vi "PH_OceanOpticsSpectrometer.PC Set Integration Time.vi"(0 "VI in":refnum<vi>, 2 "Wanted Integration Time [ms]":u16, 5 "error in (no error)":errorcluster) -> (14 "VI out":refnum<vi>, 19 "error out":errorcluster)   [LabVIEW 2014, in "PH_OceanOpticsSpectrometer.lvlib"]
doc: "This VI sets the integration time."
uses:
  PH_OceanOpticsSpectrometer.lvlib
  CS_Core/BaseProcess/BaseProcess.lvlib
  PH_Basics/PH_Common/PH_Common.lvlib
  instr.lib/OceanOpticsSpectrometer/Ocean Optics 2000 4000 - Driver np.lvlib
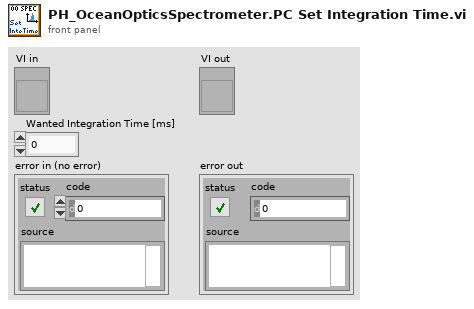
[diagram p1: front panel]
types:
  T1 = typedef "PH_OceanOpticsSpectrometer.lvlib/PH_OceanOpticsSpectrometer.i attribute.ctl" = cluster{"GUI Refs":cluster{"Delete":refnum<vi>, "Spectrum":refnum<vi>, "Display Width":refnum<vi>, "Display Center":refnum<vi>, "Save":refnum<vi>, "Integration time":refnum<vi>, "center wavelength":refnum<vi>, "width":refnum<vi>, "Wanted Trigger Mode":refnum<vi>, "Current Trigger Mode":refnum<vi>, "Trigger Info":refnum<vi>, "Model":refnum<vi>, "Driver":refnum<vi>, "Firmware":refnum<vi>}, "Display":cluster{"Width":dbl, "Center":dbl}, "VISA resource name":refnum<visa-resource-name>, "Integration time [ms]":cluster{"Current Value":u16, "Wanted Value":u16}, "Trigger":cluster{"Current value":T2, "Wanted value":T2}, "Default VISA Timeout":u32, "Last Data":cluster{"Wavelength Bins":dbl[], "Spectrum by Pixels":dbl[]}}
  T2 = typedef "PH_OceanOpticsSpectrometer.lvlib/PH_OceanOpticsSpectrometer.Trigger.ctl" = enum32{"External", "Normal"}
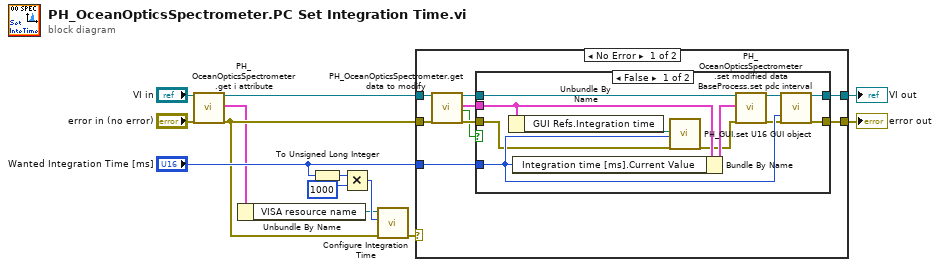
[diagram p0: block diagram]
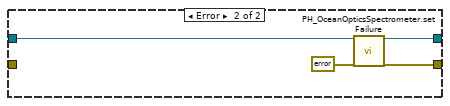
[diagram p3: hidden frame]
diagram:
  n1 = call "PH_OceanOpticsSpectrometer.get i attribute.vi"("i ref in"="VI in", "error in (no error)"="error in (no error)") -> ("i ref out"=w3:refnum<vi>, "i attribute"=w2:T1, "error out"=w5:errorcluster)  [unwired: 15 in]
  n2 = Unbundle By Name(w2) -> ("VISA resource name"=w1:refnum<visa-resource-name>)
  n3 = To Unsigned Long Integer(number="Wanted Integration Time [ms]") -> (unsigned 32bit integer=w13:u32)
  n4 = Multiply(x=w13, y=u32 1000 ("x")) -> (x*y=w9:u32)
  n5 = call "Configure Integration Time.vi"("error in (no error)"=w5, "Integration Time (6000)"=w9, "VISA resource name"=w1) -> ("error out"=w11:errorcluster)  [unwired: 7 in, 1 out]
  n6 = case shown="No Error" w11 {
    tunnel: [w22 w37] -> w7
    tunnel: w5 -> [w16 _]
    tunnel: w3 -> [w18 w39]
    tunnel: [w17 w38] -> w8
    tunnel: "Wanted Integration Time [ms]" -> [w21 _]
    frame No Error {
      n7 = call "PH_OceanOpticsSpectrometer.get data to modify.vi"("i ref in"=w18, "error in (no error)"=w16) -> ("i ref out"=w20:refnum<vi>, "i attribute"=w14:T1, "timed out"=w15:bool, "error out"=w19:errorcluster)  [unwired: 14 in]
      n8 = case shown="False" w15 {
        tunnel: [w29 w34] -> w22
        tunnel: w21 -> [w27 _]
        tunnel: w20 -> [w33 w35]
        tunnel: w19 -> [w25 w34]
        tunnel: [w30 w35] -> w17
        tunnel: w14 -> [w28 _]
        frame False {
          n9 = Unbundle By Name(w28) -> ("GUI Refs.Integration time"=w24:refnum<vi>)
          n10 = Bundle By Name(cluster=w28, "Integration time [ms].Current Value"=w27) -> (w32:T1)
          n11 = call "PH_GUI.set U16 GUI object.vi"("U16 Ref"=w24, "Value"=w27, "error in (no error)"=w25) -> ("error out"=w26:errorcluster)  [unwired: 16 in]
          n12 = call "PH_OceanOpticsSpectrometer.set modified data.vi"("i ref in"=w33, "i attribute"=w32, "error in (no error)"=w26) -> ("i ref out"=w31:refnum<vi>, "error out"=w23:errorcluster)  [unwired: 15 in]
          n13 = call "BaseProcess.set pdc interval.vi"("i ref in"=w31, "PeriodicInterval [ms]"=w27, "error in (no error)"=w23) -> ("i ref out"=w30:refnum<vi>, "error out"=w29:errorcluster)  [unwired: 14 in, 1 out]
        }
        frame True {
        }
      }
    }
    frame Error {
      n14 = call "PH_OceanOpticsSpectrometer.set Failure.vi"("i ref in"=w39, "error IO"=errorcluster {"status"=FALSE, "code"=0, "source"=""}) -> ("i ref out"=w38:refnum<vi>, "error out"=w37:errorcluster)  [unwired: 16 in]
    }
  }
  "VI out" <- w8
  "error out" <- w7
